vi "channel.vi"(8 "error in":errorcluster caption="errorIn", 11 "xmlRef":refnum<k20>) -> (0 "error out":errorcluster caption="errorOut", 3 "channels":T1[](array[typedef]))   [LabVIEW 2017]
uses:
  models/ACQ_channel.ctl
  <vilib>/xml/Close Reference(Node).vi
  <vilib>/xml/Close Reference(NdList).vi
  <resource>/objmgr/DOMUserDefRef.rc
  <vilib>/xml/NI_XML.lvlib
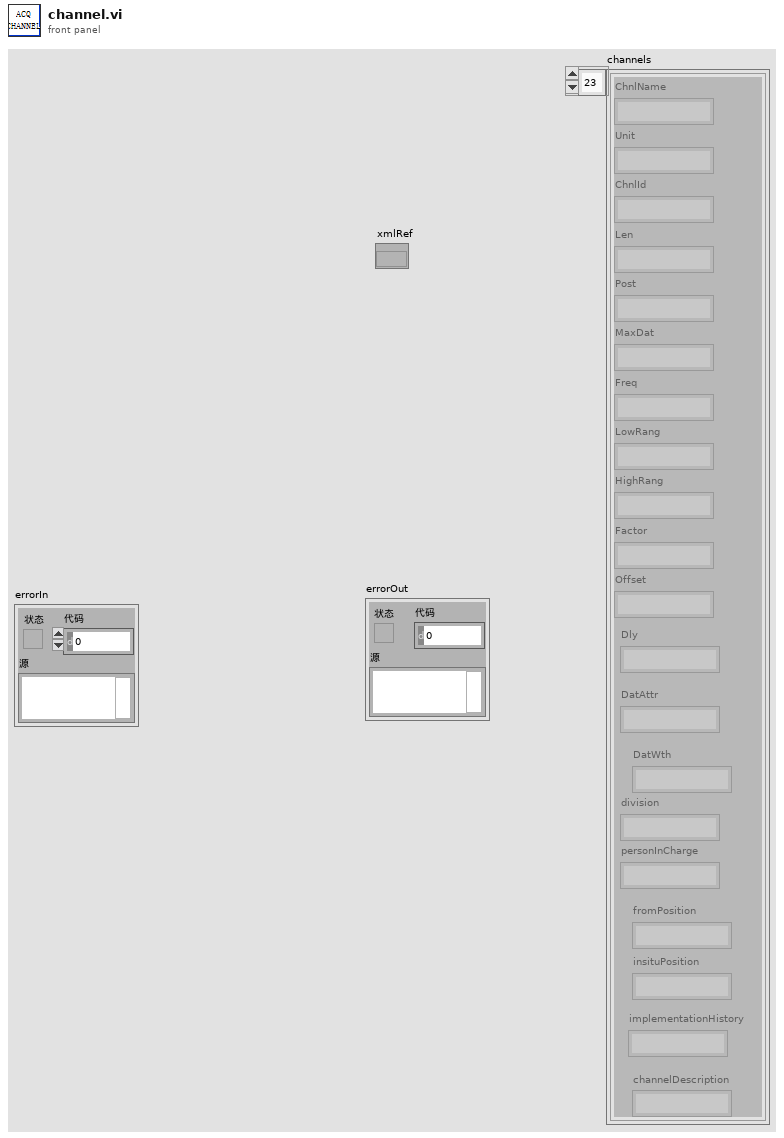
[diagram p1: front panel]
types:
  T1 = typedef "ACQ_channel.ctl" = cluster{"ChnlName":string, "Unit":string, "ChnlId":string, "Len":string, "Post":string, "MaxDat":string, "Freq":string, "LowRang":string, "HighRang":string, "Factor":string, "Offset":string, "Dly":string, "DatAttr":string, "DatWth":string, "division":string, "personInCharge":string, "fromPosition":string, "insituPosition":string, "implementationHistory":string, "channelDescription":string}
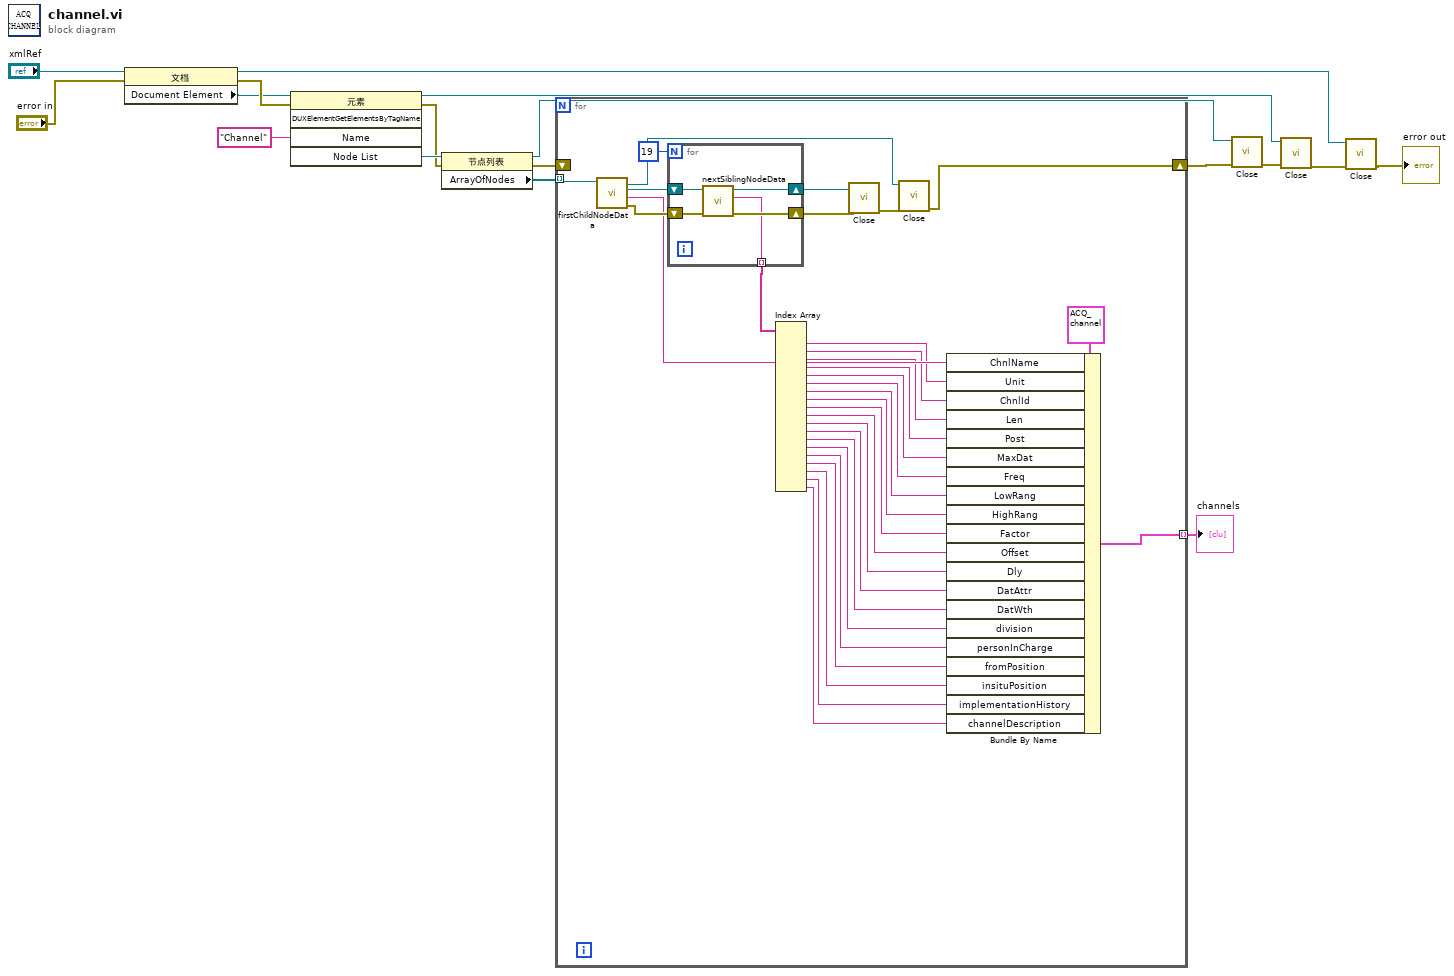
[diagram p0: block diagram]
diagram:
  n1 = property class="文档"(reference="xmlRef", error in="error in") -> (reference out=w2:refnum<k20>, error out=w16:errorcluster, "Document Element"=w15:refnum<k20>)
  n2 = invoke class="元素" method="DUXElementGetElementsByTagName"(reference=w15, error in=w16, "Name"="Channel" ("Node Name")) -> (reference out=w9:refnum<k20>, error out=w7:errorcluster, "Node List"=w8:refnum<k20>)  [unwired: 2 in, 2 out]
  n3 = property class="节点列表"(reference=w8, error in=w7) -> (reference out=w12:refnum<k20>, error out=w13:errorcluster, "ArrayOfNodes"=w14:refnum<k20>[])
  n4 = for {
    tunnel: w14 -> [w49] mode=indexing
    shift-right: [w42] -> w10
    shift-left: w13 -> [_]
    tunnel: [w20] -> w1 mode=indexing
    n5 = call "firstChildNodeData.vi"("parentNode"=w49) -> ("error out"=w47:errorcluster, "data"=w39:string, "childNode"=w48:refnum<k20>, "parentNode"=w43:refnum<k20>)  [unwired: 7 in]
    n6 = for {
      N: 19 -> [_]
      shift-right: [w53] -> w46
      shift-left: w48 -> [w54]
      tunnel: [w50] -> w41 mode=indexing
      shift-right: [w51] -> w45
      shift-left: w47 -> [w52]
      n7 = call "nextSiblingNodeData.vi"("error in (no error)"=w52, "siblingNode"=w54) -> ("error out"=w51:errorcluster, "data"=w50:string, "childNode"=w53:refnum<k20>)  [unwired: 7 in]
    }
    n8 = Index Array(array=w41) -> (element #1=w38:string, element #2=w37:string, element #3=w36:string, element #4=w35:string, element #5=w34:string, element #6=w33:string, element #7=w32:string, element #8=w31:string, element #9=w30:string, element #10=w29:string, element #11=w28:string, element #12=w27:string, element #13=w26:string, element #14=w25:string, element #15=w24:string, element #16=w23:string, element #17=w22:string, element #18=w21:string, element #19=w18:string)  [unwired: 19 in]
    n9 = call-poly <vilib>:"Close.vi"("error in (no error)"=w45, "node"=w46) -> ("error out"=w44:errorcluster)  [unwired: 7 out]
    n10 = call-poly <vilib>:"Close.vi"("error in (no error)"=w44, "node"=w43) -> ("error out"=w42:errorcluster)  [unwired: 7 out]
    n11 = Bundle By Name(cluster=T1 {"ChnlName"="", "Unit"="", "ChnlId"="", "Len"="", "Post"="", "MaxDat"="", "Freq"="", "LowRang"="", "HighRang"="", "Factor"="", "Offset"="", "Dly"="", "DatAttr"="", "DatWth"="", "division"="", "personInCharge"="", "fromPosition"="", "insituPosition"="", "implementationHistory"="", "channelDescription"=""} ("channel"), "ChnlName"=w39, "Unit"=w38, "ChnlId"=w37, "Len"=w36, "Post"=w35, "MaxDat"=w34, "Freq"=w33, "LowRang"=w32, "HighRang"=w31, "Factor"=w30, "Offset"=w29, "Dly"=w28, "DatAttr"=w27, "DatWth"=w26, "division"=w25, "personInCharge"=w24, "fromPosition"=w23, "insituPosition"=w22, "implementationHistory"=w21, "channelDescription"=w18) -> (w20:T1)
  }
  "channels" <- w1
  n12 = call-poly <vilib>:"Close.vi"("error in (no error)"=w10, "node list"=w12) -> ("error out"=w11:errorcluster)  [unwired: 7 out]
  n13 = call-poly <vilib>:"Close.vi"("error in (no error)"=w11, "node"=w9) -> ("error out"=w4:errorcluster)  [unwired: 7 out]
  n14 = call-poly <vilib>:"Close.vi"("error in (no error)"=w4, "node"=w2) -> ("error out"=→"error out":errorcluster)  [unwired: 7 out]
